vi "fgv buffer image references.vi"(0 "Image Reference IN":T3, 1 "Actions":T4, 5 "Imaging Parameters":T1, 9 "Calibration Parameters":T2, 11 "error in (no error)":errorcluster, 12 "index(s)":i32[](array[numeric]), 13 "element":string) -> (3 "Imag ref. name":string[](array[string]), 4 "Image Array":T3[](array[typedef]), 6 "LB data":string[][](array[string]), 8 "Imaging Parameters":T1[](array[typedef]), 10 "Calibration Parameters":T2[](array[typedef]), 14 "LB data full":string[][](array[string]), 15 "error out":errorcluster)   [LabVIEW 2020]
uses:
  ToolBox/TypeDefs/data and image buffer fgv actions.ctl
  <vilib>/vision/Image Controls.llb/IMAQ Image.ctl
  ToolBox/TypeDefs/Current Calibration Parameters.ctl
  ToolBox/TypeDefs/Current Imaging Parameters.ctl
  138bf972-3e2c-4b9c-869a-8880fb0fa013.vi
  34bb193f-b545-427e-b1e4-c07e80b324ef.vi
  f5771faa-6821-441f-a328-0f121c78e6d9.vi
  d3480d6e-a209-486d-a997-ed0cab6325bc.vi
  <vilib>/Analysis/1siggen.llb/Ramp Pattern by Samples.vi
  <vilib>/Analysis/NI_AALBase.lvlib
panel:
  out "Sr No.":i32[](array[numeric])
  # "Note elements and index(s) are multi-use"
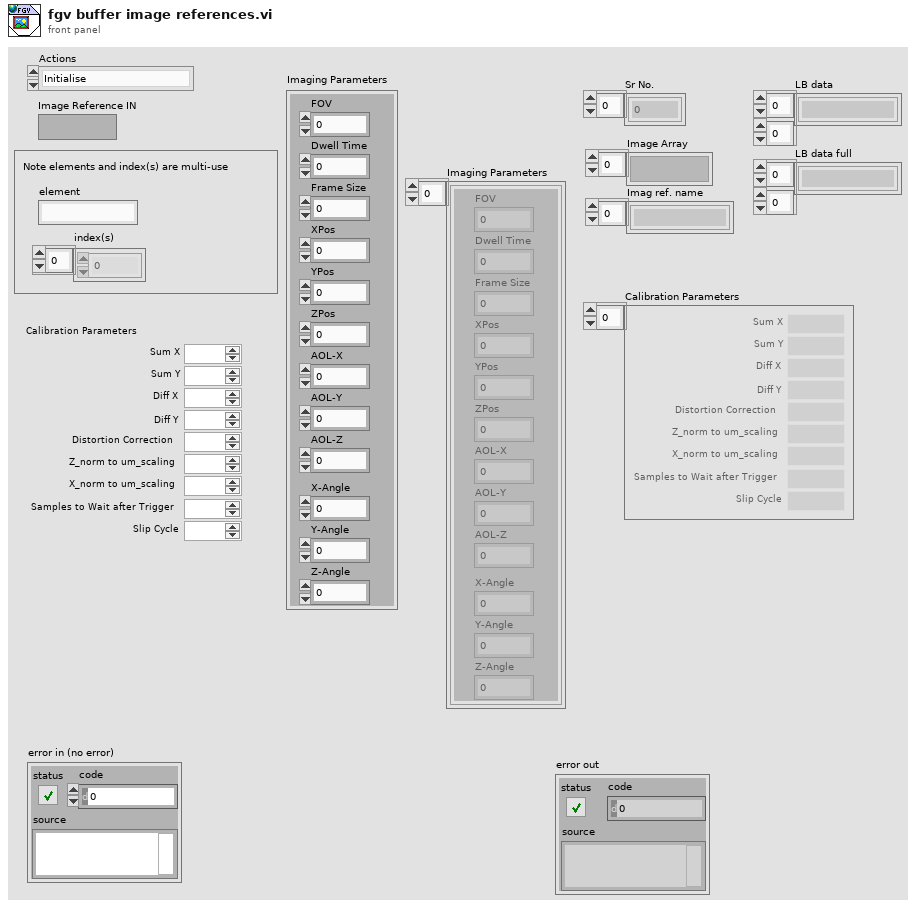
[diagram p1: front panel]
types:
  T1 = typedef "Current Imaging Parameters.ctl" = cluster{"FOV":dbl, "Dwell Time":dbl, "Frame Size":dbl, "XPos":dbl, "YPos":dbl, "ZPos":dbl, "AOL-X":dbl, "AOL-Y":dbl, "AOL-Z":dbl, "X-Angle":dbl, "Y-Angle":dbl, "Z-Angle":dbl}
  T2 = typedef "Current Calibration Parameters.ctl" = cluster{"Sum X":dbl, "Sum Y":dbl, "Diff X":dbl, "Diff Y":dbl, "Distortion Correction":dbl, "Z_norm to um_scaling":dbl, "X_norm to um_scaling":dbl, "Samples to Wait after Trigger":dbl, "Slip Cycle":dbl}
  T3 = typedef "IMAQ Image.ctl" = refnum<image>
  T4 = typedef "data and image buffer fgv actions.ctl" = enum16{"Initialise", "Add Image to buffer", "Read Image buffer", "Edit specific data", "Delete selected image", "Clear all images"}
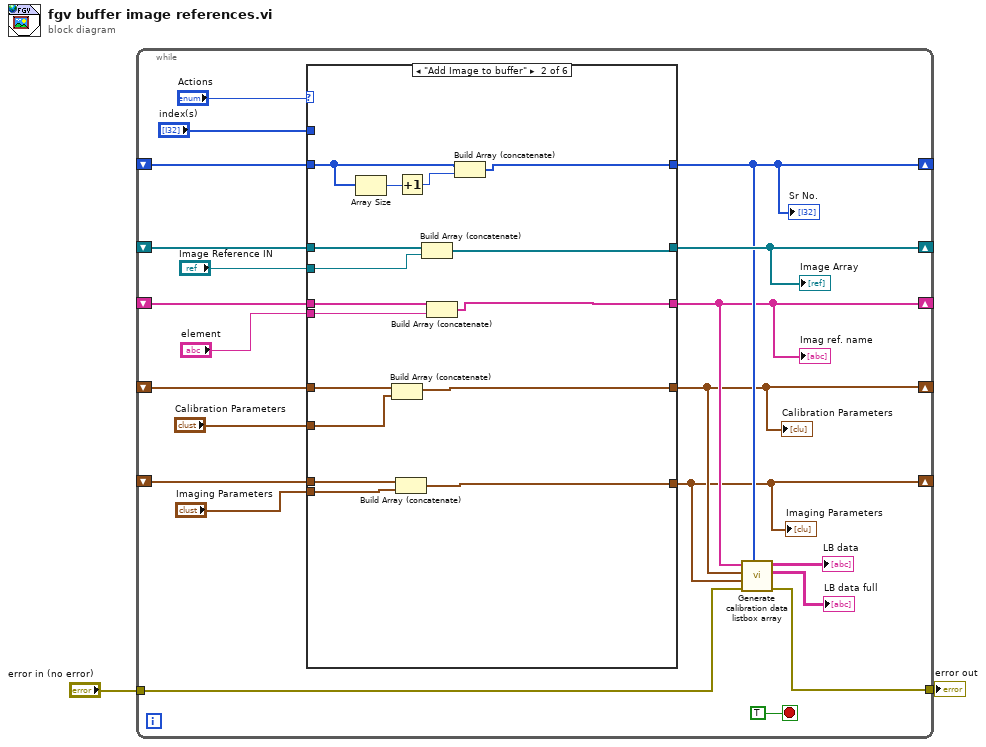
[diagram p0: block diagram]
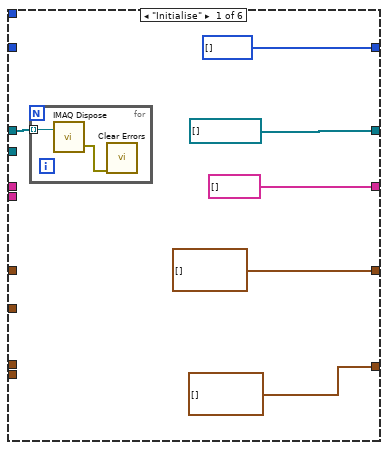
[diagram p2: hidden frame]
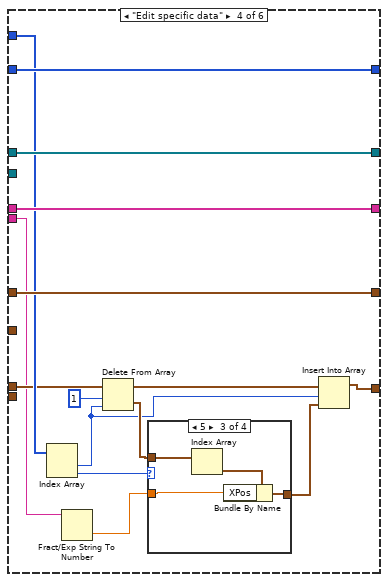
[diagram p4: hidden frame]
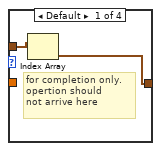
[diagram p5: hidden frame]
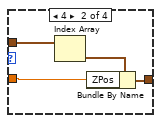
[diagram p6: hidden frame]
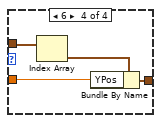
[diagram p7: hidden frame]
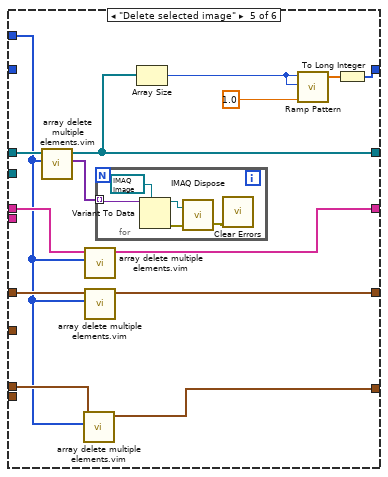
[diagram p8: hidden frame]
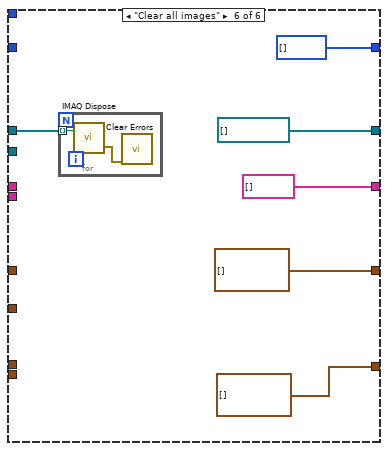
[diagram p9: hidden frame]
diagram:
  n1 = while {
    shift-right: [w22] -> _
    shift-left: _ -> [w21]
    tunnel: "error in (no error)" -> [w6]
    tunnel: [w5] -> w1
    shift-right: [w8] -> _
    shift-left: _ -> [w19]
    shift-right: [w7] -> _
    shift-left: _ -> [w17]
    shift-right: [w9] -> _
    shift-left: _ -> [w15]
    shift-right: [w10] -> _
    shift-left: _ -> [w11]
    stop <- TRUE stop-if-true
    n2 = case shown="\"Add Image to buffer\"" "Actions" {
      tunnel: [T3[] [] ("RedImageArray") w46 w52 w66 w87 T3[] [] ("RedImageArray")] -> w22
      tunnel: w21 -> [w28 w47 w52 w66 w91 w106]
      tunnel: "index(s)" -> [_ _ _ w63 w83 _]
      tunnel: [T2[] [] w32 w51 w64 w94 T2[] []] -> w8
      tunnel: w19 -> [_ w45 w51 w64 w95 _]
      tunnel: "Calibration Parameters" -> [_ w44 _ _ _ _]
      tunnel: [T1[] [] w34 w50 w53 w92 T1[] []] -> w7
      tunnel: w17 -> [_ w43 w50 w62 w93 _]
      tunnel: "Imaging Parameters" -> [_ w42 _ _ _ _]
      tunnel: [string[] [] w33 w48 w65 w82 string[] []] -> w9
      tunnel: w15 -> [_ w41 w48 w65 w84 _]
      tunnel: "element" -> [_ w40 _ w58 _ _]
      tunnel: [i32[] [] w35 w49 w67 w85 i32[] []] -> w10
      tunnel: "Image Reference IN" -> [_ w39 _ _ _ _]
      tunnel: w11 -> [_ w37 w49 w67 _ _]
      frame "Initialise" {
        n3 = for {
          tunnel: w28 -> [w31] mode=indexing
          n4 = call "IMAQ Dispose"("Image"=w31) -> ("error out"=w30:errorcluster)  [unwired: 5 in]
          n5 = call <vilib>:"Clear Errors.vi"("error in (no error)"=w30) -> ()  [unwired: 5 in, 2 out]
        }
      }
      frame "Add Image to buffer" {
        n6 = Array Size(array=w37) -> (size(s)=w38:i32)
        n7 = Build Array (concatenate)(w45, w44) -> (w32:T2[])
        n8 = Build Array (concatenate)(w43, w42) -> (w34:T1[])
        n9 = Increment(x=w38) -> (x+1=w36:i32)
        n10 = Build Array (concatenate)(w47, w39) -> (w46:T3[])
        n11 = Build Array (concatenate)(w41, w40) -> (w33:string[])
        n12 = Build Array (concatenate)(w37, w36) -> (w35:i32[])
      }
      frame "Read Image buffer" {
      }
      frame "Edit specific data" {
        n13 = Index Array(array=w63) -> (element #1=w56:i32, element #2=w60:i32)  [unwired: 2 in]
        n14 = Fract/Exp String To Number(string=w58) -> (number=w57:dbl)  [unwired: 3 in, 1 out]
        n15 = Delete From Array(array=w62, length=1, index=w56) -> (deleted portion=w59:T1[], array with subset deleted=w55:T1[])
        n16 = case shown="5" w60 {
          tunnel: w59 -> [w69 w72 w76 w81]
          tunnel: w57 -> [_ w71 w75 w79]
          tunnel: [w68 w70 w74 w78] -> w54
          frame Default {
            # "for completion only.\nopertion should \nnot arrive here"
            n17 = Index Array(array=w69) -> (element=w68:T1)  [unwired: 1 in]
          }
          frame 4 {
            n18 = Index Array(array=w72) -> (element=w73:T1)  [unwired: 1 in]
            n19 = Bundle By Name(cluster=w73, "ZPos"=w71) -> (w70:T1)
          }
          frame 5 {
            n20 = Index Array(array=w76) -> (element=w77:T1)  [unwired: 1 in]
            n21 = Bundle By Name(cluster=w77, "XPos"=w75) -> (w74:T1)
          }
          frame 6 {
            n22 = Index Array(array=w81) -> (element=w80:T1)  [unwired: 1 in]
            n23 = Bundle By Name(cluster=w80, "YPos"=w79) -> (w78:T1)
          }
        }
        n24 = Insert Into Array(array=w55, index=w56, new element=w54) -> (w53:T1[])
      }
      frame "Delete selected image" {
        n25 = call "array delete multiple elements.vim"("Index(s)"=w83, "1D Array IN"=w91) -> ("Deleted Elemets"=w90:variant[], "1D Array OUT"=w87:T3[])  [unwired: 7 in, 1 out]
        n26 = call "array delete multiple elements.vim"("Index(s)"=w83, "1D Array IN"=w93) -> ("1D Array OUT"=w92:T1[])  [unwired: 7 in, 2 out]
        n27 = call "array delete multiple elements.vim"("Index(s)"=w83, "1D Array IN"=w84) -> ("1D Array OUT"=w82:string[])  [unwired: 7 in, 2 out]
        n28 = call "array delete multiple elements.vim"("Index(s)"=w83, "1D Array IN"=w95) -> ("1D Array OUT"=w94:T2[])  [unwired: 7 in, 2 out]
        n29 = for {
          tunnel: w90 -> [w100] mode=indexing
          n30 = Variant To Data(type=T3 refnum ("Image"), Variant=w100) -> (data=w98:T3, error out=w97:errorcluster)  [unwired: 1 in]
          n31 = call "IMAQ Dispose"("Image"=w98, "error in (no error)"=w97) -> ("error out"=w96:errorcluster)  [unwired: 4 in]
          n32 = call <vilib>:"Clear Errors.vi"("error in (no error)"=w96) -> ()  [unwired: 5 in, 2 out]
        }
        n33 = Array Size(array=w87) -> (size(s)=w86:i32)
        n34 = call-poly <vilib>:"Ramp Pattern.vi"("start"=1.0, "end"=w86, "samples"=w86) -> ("Ramp Pattern"=w88:dbl[])  [unwired: 7 in, 1 out]
        n35 = To Long Integer(number=w88) -> (32bit integer=w85:i32[])
      }
      frame "Clear all images" {
        n36 = for {
          tunnel: w106 -> [w108] mode=indexing
          n37 = call "IMAQ Dispose"("Image"=w108) -> ("error out"=w107:errorcluster)  [unwired: 5 in]
          n38 = call <vilib>:"Clear Errors.vi"("error in (no error)"=w107) -> ()  [unwired: 5 in, 2 out]
        }
      }
    }
    "Image Array" <- w22
    "Calibration Parameters" <- w8
    "Imaging Parameters" <- w7
    "Imag ref. name" <- w9
    "Sr No." <- w10
    n39 = call "Generate calibration data listbox array .vi"("Sr No."=w10, "error in (no error)"=w6, "Imaging Parameters"=w7, "Calibration data"=w8, "Imag ref. name"=w9) -> ("error out"=w5:errorcluster, "LB data full"=→"LB data full":string[][], "LB data trunc"=→"LB data":string[][])  [unwired: 4 in]
  }
  "error out" <- w1
